vi "Normalize Angle in Degrees.vi"(11 "Angle deg":dbl) -> (3 "Angle":dbl)   [LabVIEW 2019]
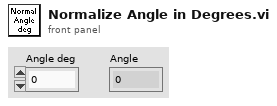
[diagram p1: front panel]
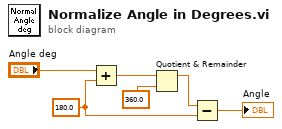
[diagram p0: block diagram]
diagram:
  w2 = 180.0
  n1 = Add(x="Angle deg", y=w2) -> (x+y=w3:dbl)
  n2 = Quotient & Remainder(x=w3, y=360.0) -> (x-y*floor(x/y)=w4:dbl)  [unwired: 1 out]
  n3 = Subtract(x=w4, y=w2) -> (x-y=→"Angle":dbl)
